vi "DeCoF open connection.vi"(4 "error in (no error)":errorcluster, 6 "TCP?":bool=TRUE, 7 "address":string) -> (0 "error out":errorcluster, 3 "Conncection ID out":T1)   [LabVIEW 2013]
doc: "Opens a connection to the remote device.\n\"Connection ID in\" can either be an ip address, if the TCP? input is set to TRUE or the VISA name of a serial port is the TCP? input is set to FALSE.\nThe \"Connection ID out\" indicator returns an ID which has to be wired to the other communication commands.\n\nThe port for TCP connections is set to 50000.\nThe baud rate for serial connections is set to 115200."
uses:
  subVIs/DeCoF connection.ctl
  <vilib>/Instr/_visa.llb/Select Event Type.ctl
  <vilib>/Instr/_visa.llb/VISA Configure Serial Port (Instr).vi
panel:
  out "welcome string":string
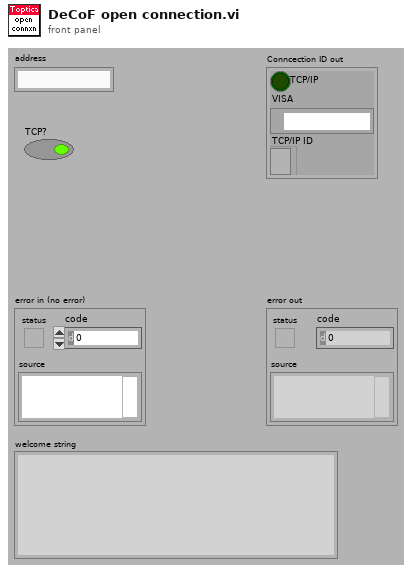
[diagram p1: front panel]
types:
  T1 = typedef "DeCoF connection.ctl" = cluster{"TCP/IP":bool, "VISA":refnum<visa-resource-name>, "TCP/IP ID":refnum<k5>}
  T2 = typedef "Select Event Type.ctl" = u32
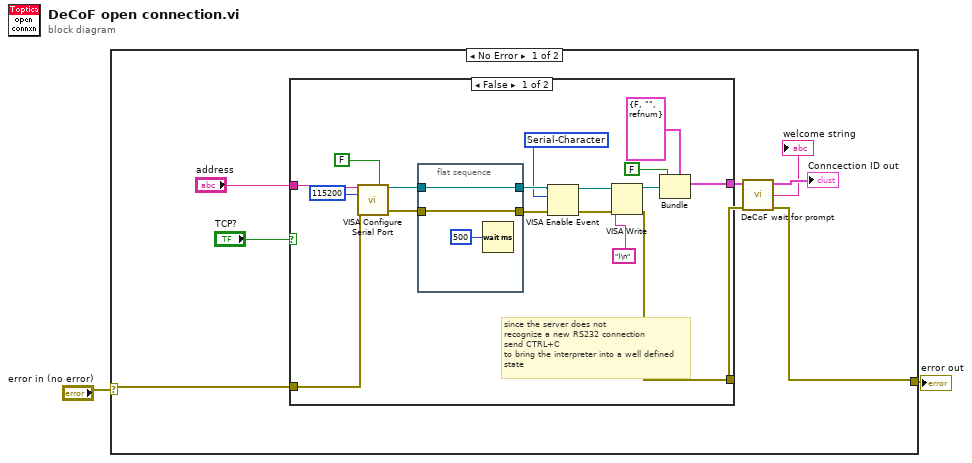
[diagram p0: block diagram]
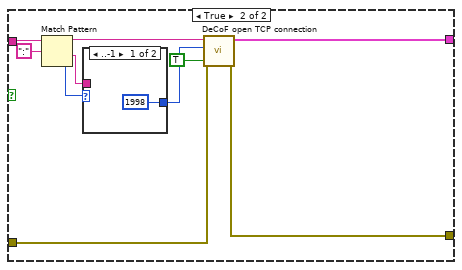
[diagram p2: hidden frame]
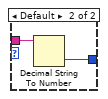
[diagram p3: hidden frame]
diagram:
  n1 = case shown="No Error" "error in (no error)" {
    selector: "error in (no error)" -> [w9 w44]
    tunnel: [w5 w44] -> w1
    frame No Error {
      n2 = case shown="False" "TCP?" {
        tunnel: "address" -> [w22 w36]
        tunnel: w9 -> [w27 w40]
        tunnel: [w23 w39] -> w4
        tunnel: [w16 w37] -> w6
        frame False {
          w13 = T2 1073684533 items=["ServiceRequest"=1073684491, "Trigger"=3221168138, "Clear"=1073684493, "VXI-Signal"=1073684512, "VXI/VME-Interrupt"=3221168161, "VXI/VME-Sysfail"=1073684509, "VXI/VME-Sysreset"=1073684510, "GPIB-CIC"=1073684498, "GPIB-Talk"=1073684499, "GPIB-Listen"=1073684500, "PXI-Interrupt"=1073684514, "Serial-Break"=1073684515, "Serial-TermChar"=1073684516, "Serial-CTS"=1073684521, "Serial-DSR"=1073684522, "Serial-DCD"=1073684524, "Serial-RI"=1073684526, "Serial-Character"=1073684533, "USB-Interrupt"=1073684535, "AllEnabled"=1073709055] ("Event Type")
          # "since the server does not\nrecognize a new RS232 connection\nsend CTRL+C\nto bring the interpreter into a well defined \nstate"
          n3 = call-poly "VISA Configure Serial Port"("VISA resource name"=w22, "Enable Termination\nChar (T)"=FALSE ("Enable Termination\nChar (T)"), "baud rate (9600)"=u32 115200, "error in (no error)"=w27) -> ("VISA resource name out"=w20:refnum<visa-resource-name>, "error out"=w21:errorcluster)  [unwired: 10 in]
          n4 = flat-sequence {
            tunnel: [w29] -> w14
            tunnel: w21 -> [w29]
            tunnel: w20 -> [w28]
            tunnel: [w28] -> w15
            frame #0 {
              n5 = Wait (ms)(milliseconds to wait=u32 500) -> ()  [unwired: 1 out]
            }
          }
          n6 = VISA Enable Event(8:w14, 10:w13, 11:w15) -> (0:w11:errorcluster, 3:w12:refnum<visa-resource-name>)  [unwired: 1 in]
          n7 = VISA Write(VISA resource name=w12, write buffer=")\n", error in (no error)=w11) -> (VISA resource name out=w18:refnum<visa-resource-name>, error out=w23:errorcluster)  [unwired: 1 out]
          n8 = Bundle(cluster=T1 {"TCP/IP"=FALSE, "VISA"="", "TCP/IP ID"=refnum} ("Conncection ID out"), "TCP/IP"=FALSE, "VISA"=w18) -> (w16:T1)  [unwired: 1 in]
        }
        frame True {
          n9 = Match Pattern(string=w36, regular expression=":") -> (before substring=w34:string, after substring=w32:string, offset past match=w33:i32)  [unwired: 1 in, 1 out]
          n10 = case shown="..-1" w33 {
            tunnel: w32 -> [_ w43]
            tunnel: [1998 w42] -> w31
            frame ..-1 {
            }
            frame Default {
              n11 = Decimal String To Number(string=w43) -> (number=w42:i32)  [unwired: 2 in, 1 out]
            }
          }
          n12 = call "DeCoF open TCP connection.vi"("error in (no error)"=w40, "TCP_NODELAY (true)"=TRUE, "remote port"=w31, "address"=w34) -> ("error out"=w39:errorcluster, "TCP Connection ID"=w37:T1)  [unwired: 2 in]
        }
      }
      n13 = call "DeCoF wait for prompt.vi"("Connection ID in"=w6, "error in (no error)"=w4) -> ("complete answer"=→"welcome string":string, "Conncection ID out"=→"Conncection ID out":T1, "error out"=w5:errorcluster)  [unwired: 2 in, 2 out]
    }
    frame Error {
    }
  }
  "error out" <- w1
